vi "Test Vectors (MD5).vi"() -> (3 "All Vectors passed":bool)   [LabVIEW 2013]
uses:
  MD5.lvclass
  MD5.lvlib
panel:
  out "1 million character message":bool
  out "String tests":bool[](array[boolean])
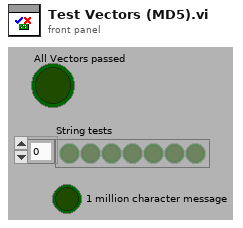
[diagram p1: front panel]
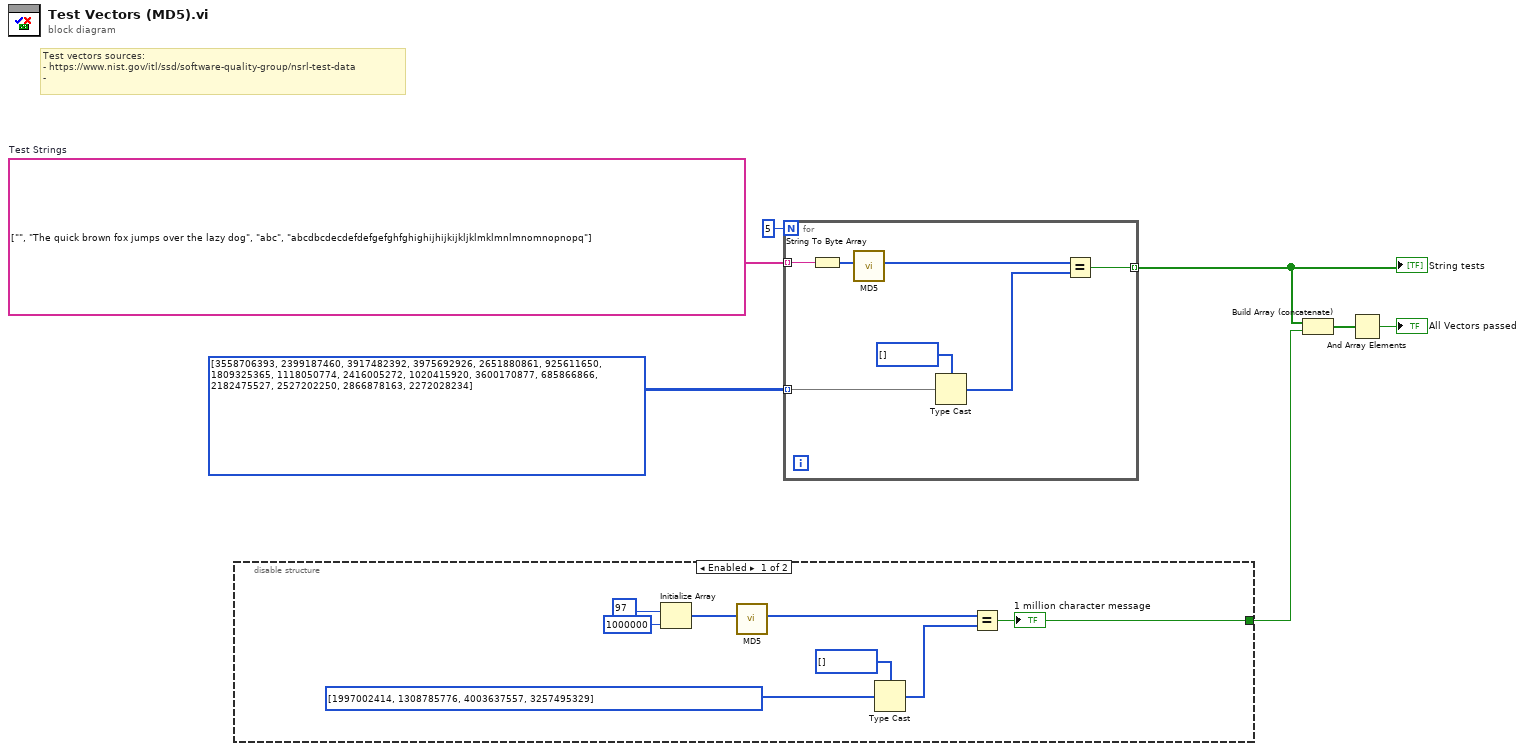
[diagram p0: block diagram]
diagram:
  w7 = string[] ["", "The quick brown fox jumps over the lazy dog", "abc", "abcdbcdecdefdefgefghfghighijhijkijkljklmklmnlmnomnopnopq"]  # Test Strings
  # "Test vectors sources:\n- https://www.nist.gov/itl/ssd/software-quality-group/nsrl-test-data\n-"
  n1 = disable-structure shown="Enabled" {
    disable-tunnel: [w8 _] -> w5
    frame Enabled {
      n2 = Initialize Array(u8 97 ("Numeric"), 1000000 ("dimension size")) -> (w13:u8[])
      n3 = call "MD5.vi"("data"=w13) -> ("MD5 hash"=w12:u8[])  [unwired: 10 in]
      n4 = Type Cast(type=u8[] [], x=u32[] [1997002414, 1308785776, 4003637557, 3257495329]) -> (*(type *) &x=w9:u8[])
      n5 = Equal?(x=w12, y=w9) -> (x = y?=w8:bool)
      "1 million character message" <- w8
    }
    frame Disabled {
    }
  }
  n6 = for {
    N: 5 -> [_]
    tunnel: w7 -> [w22] mode=indexing
    tunnel: u32[][] [[3558706393, 2399187460, 3917482392, 3975692926], [2651880861, 925611650, 1809325365, 1118050774], [2416005272, 1020415920, 3600170877, 685866866], [2182475527, 2527202250, 2866878163, 2272028234]] -> [w17] mode=indexing
    tunnel: [w21] -> w6 mode=indexing
    n7 = String To Byte Array(string=w22) -> (unsigned byte array=w20:u8[])
    n8 = call "MD5.vi"("data"=w20) -> ("MD5 hash"=w19:u8[])  [unwired: 10 in]
    n9 = Type Cast(type=u8[] [], x=w17) -> (*(type *) &x=w16:u8[])
    n10 = Equal?(x=w19, y=w16) -> (x = y?=w21:bool)
  }
  "String tests" <- w6
  n11 = Build Array (concatenate)(w6, w5) -> (w4:bool[])
  n12 = And Array Elements(Boolean array=w4) -> (logical AND=→"All Vectors passed":bool)
